vi "create_files.vi"(9 "log data cluster":T1, 10 "start?":bool, 11 "base path":path) -> ()   [LabVIEW 2019]
uses:
  typedefs/log_data_cluster.ctl
  <vilib>/Utility/file.llb/Write Delimited Spreadsheet (DBL).vi
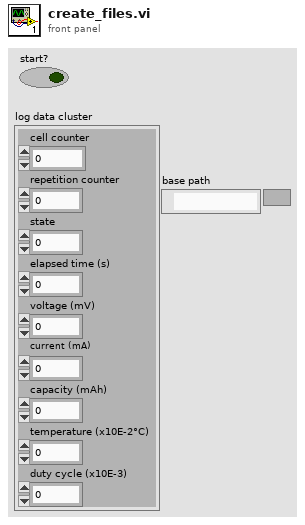
[diagram p1: front panel]
types:
  T1 = typedef "log_data_cluster.ctl" = cluster{"cell counter":u8, "repetition counter":u8, "state":u8, "elapsed time (s)":u16, "voltage (mV)":u16, "current (mA)":u16, "capacity (mAh)":u16, "temperature (x10E-2°C)":u16, "duty cycle (x10E-3)":u16}
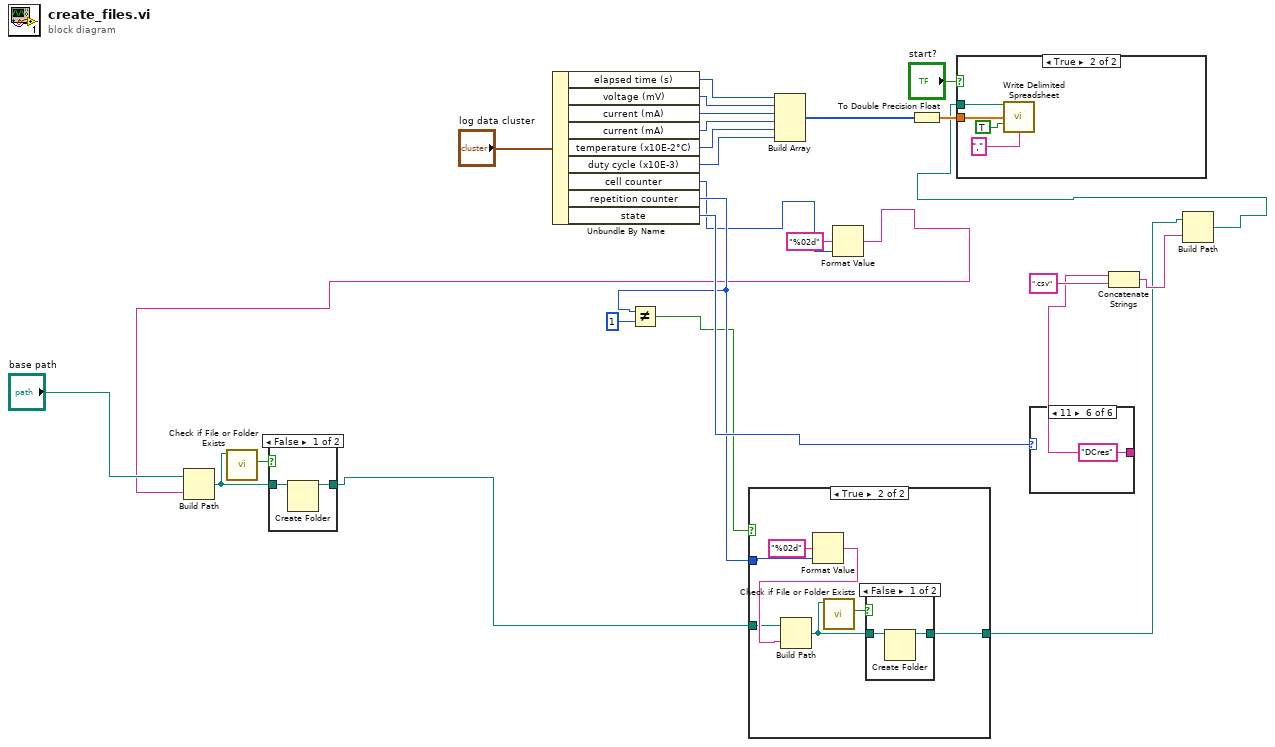
[diagram p0: block diagram]
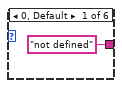
[diagram p5: hidden frame]
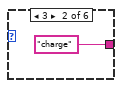
[diagram p6: hidden frame]
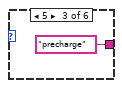
[diagram p7: hidden frame]
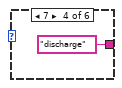
[diagram p8: hidden frame]
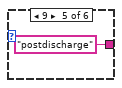
[diagram p9: hidden frame]
diagram:
  n1 = Unbundle By Name("log data cluster") -> ("elapsed time (s)"=w17:u16, "voltage (mV)"=w18:u16, "current (mA)"=w19:u16, "current (mA)"=w20:u16, "temperature (x10E-2°C)"=w21:u16, "duty cycle (x10E-3)"=w22:u16, "cell counter"=w11:u8, "repetition counter"=w15:u8, "state"=w16:u8)
  n2 = Not Equal?(x=w15, y=u8 1) -> (x != y?=w13:bool)
  n3 = Build Array(w17, w18, w19, w20, w21, w22) -> (w23:u16[])
  n4 = Format Value(format string="%02d", value (0)=w11) -> (output string=w5:string)  [unwired: 1 in]
  n5 = Build Path(base path="base path", name or relative path=w5) -> (appended path=w8:path)
  n6 = call <vilib>:"Check if File or Folder Exists.vi"("path"=w8) -> ("file or folder exists?"=w7:bool)  [unwired: 8 in, 2 out]
  n7 = case shown="False" w7 {
    tunnel: [w27 w29] -> w4
    tunnel: w8 -> [w28 w29]
    frame False {
      n8 = Create Folder(path (use dialog)=w28) -> (created path=w27:path)  [unwired: 2 in, 2 out]
    }
    frame True {
    }
  }
  n9 = case shown="True" w13 {
    tunnel: w15 -> [_ w36]
    tunnel: w4 -> [w30 w32]
    tunnel: [w30 w31] -> w1
    frame False {
    }
    frame True {
      n10 = Format Value(format string="%02d", value (0)=w36) -> (output string=w33:string)  [unwired: 1 in]
      n11 = Build Path(base path=w32, name or relative path=w33) -> (appended path=w35:path)
      n12 = call <vilib>:"Check if File or Folder Exists.vi"("path"=w35) -> ("file or folder exists?"=w34:bool)  [unwired: 8 in, 2 out]
      n13 = case shown="False" w34 {
        tunnel: [w38 w40] -> w31
        tunnel: w35 -> [w39 w40]
        frame False {
          n14 = Create Folder(path (use dialog)=w39) -> (created path=w38:path)  [unwired: 2 in, 2 out]
        }
        frame True {
        }
      }
    }
  }
  n15 = To Double Precision Float(number=w23) -> (double precision float=w24:dbl[])
  n16 = case shown="11" w16 {
    tunnel: ["not defined" "charge" "precharge" "discharge" "postdischarge" "DCres"] -> w2
    frame 0, Default {
    }
    frame 3 {
    }
    frame 5 {
    }
    frame 7 {
    }
    frame 9 {
    }
    frame 11 {
    }
  }
  n17 = Concatenate Strings(w2, ".csv" ("string")) -> (w12:string)
  n18 = Build Path(base path=w1, name or relative path=w12) -> (appended path=w9:path)
  n19 = case shown="True" "start?" {
    tunnel: w24 -> [_ w50]
    tunnel: w9 -> [_ w47]
    frame False {
    }
    frame True {
      n20 = call-poly <vilib>:"Write Delimited Spreadsheet.vi"("file path (dialog if empty)"=w47, "1D data"=w50, "append to file? (new file:F)"=TRUE, "delimiter (\\t)"="," ("delimiter (\\t)")) -> ()  [unwired: 10 in, 2 out]
    }
  }
